vi "Polarization_Simulation.vi"() -> ()   [LabVIEW 2018]
panel:
  in  "Drive Zero Level Down":bool
  in  "Thermally Connect Zero Ensemble":bool
  in  "Zero Ensemble Power":dbl=0.05
  in  "Zero Lorentzian Position":dbl=1.0
  in  "Zero Lorentzian Width":dbl=0.05
  in  "Zero Ensemble Area":dbl=0.1
  in  "Zero Level on":bool
  in  "Gaussian Noise SD":dbl
  in  "AFP Efficiency":dbl=0.8
  in  "Timing (ms)":i32=10
  out "XY Graph 3":cluster{dbl[], "rho- out":dbl[]}[](graph)
  in  "AFP Sweep Direction":u16(ring) items=["Positive", "Negative"]
  in  "RF Proportional to Intensity":bool
  in  "File operation":u16(ring) items=["Open existing file", "Create new file", "Replace existing file"]
  out "XY Graph 2":cluster{"Array":dbl[], "Array 2":dbl[]}(graph)
  in  "Sweep AFP Range":bool
  in  "RF Power":dbl=0.1 min=0.0 max=1.0 step=0.01
  in  "Also use RF Range 2":bool
  in  "RF on":bool
  out "XY Graph":cluster{dbl[], "rho+ array out":dbl[]}[](graph)
  in  "Microwave on":bool
  in  "AFP Slider":cluster{i32, i32}(slide)={0, 500} scale=0.0..500.0
  in  "RF Slider 2":cluster{i32, i32}(slide)={0, 4} scale=0.0..500.0
  in  "RF Slider 1":cluster{i32, i32}(slide)={201, 238} scale=0.0..500.0
  in  "Relaxation Rate":dbl min=0.0 max=1.0 step=0.0001
  in  "Microwave Power":dbl=0.05 min=0.0 max=1.0 step=0.001
  in  "Saturation Polarization":dbl=0.45 min=0.0 max=0.99 step=0.01
  in  "Signal Lorentzian Width":dbl=0.005 min=0.0 step=0.001
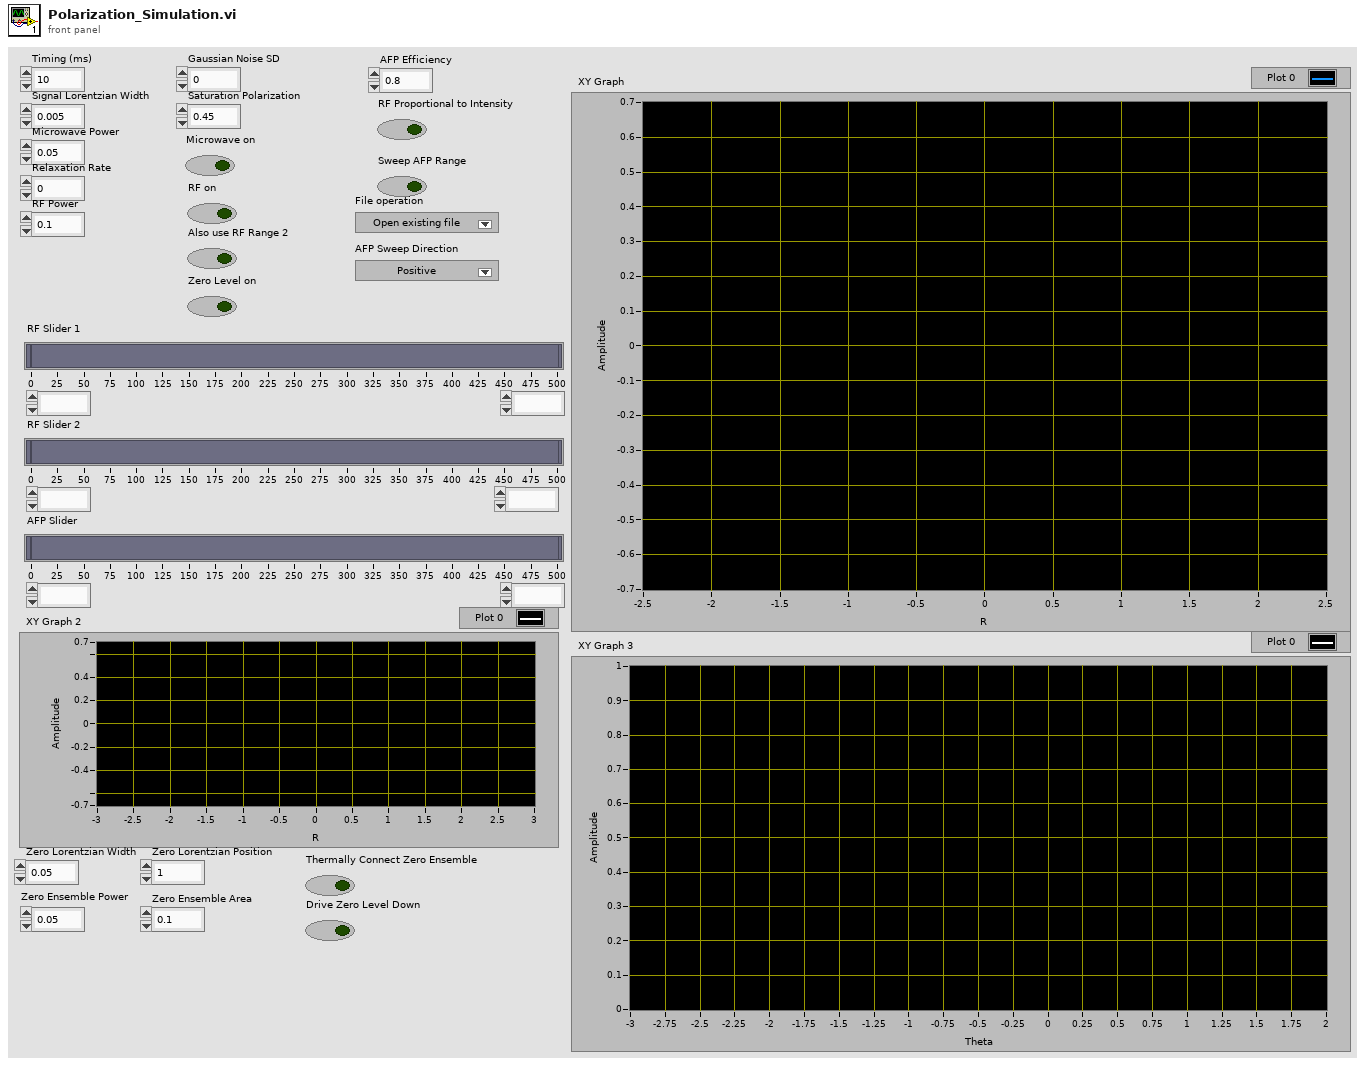
[diagram p1: front panel]
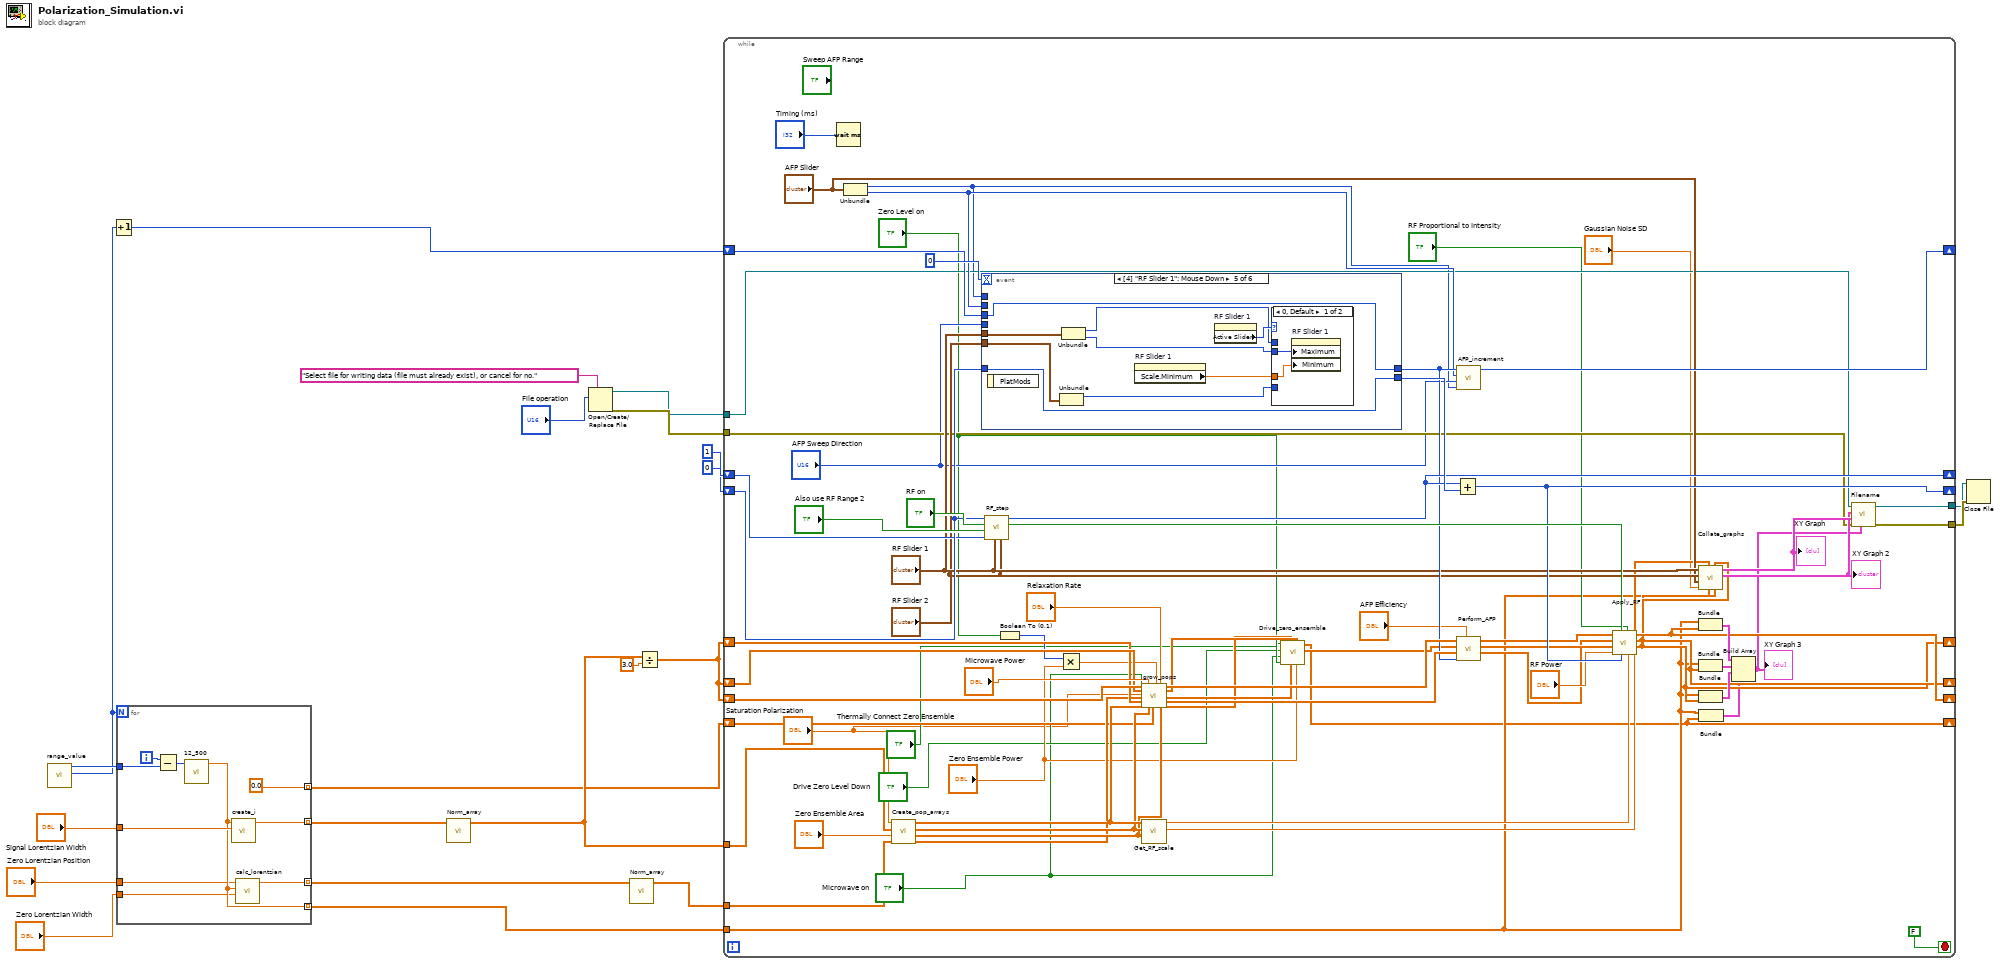
[diagram p0: block diagram]
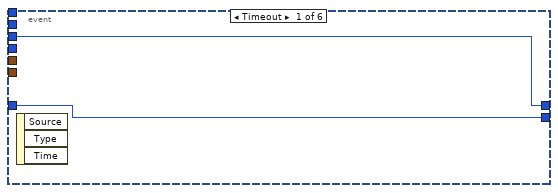
[diagram p2: hidden frame]
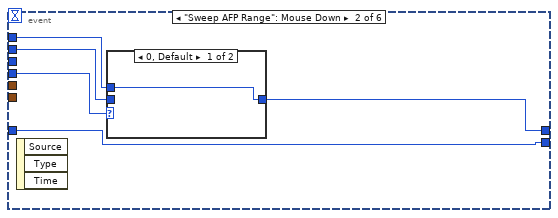
[diagram p3: hidden frame]
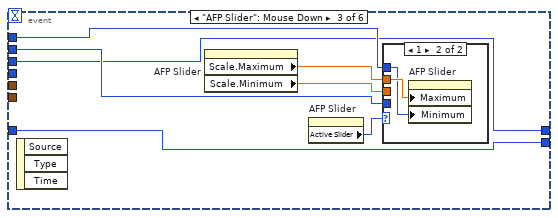
[diagram p5: hidden frame]
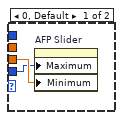
[diagram p6: hidden frame]
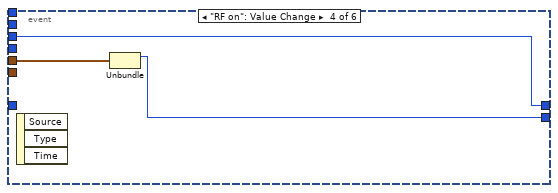
[diagram p7: hidden frame]
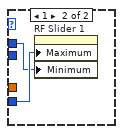
[diagram p8: hidden frame]
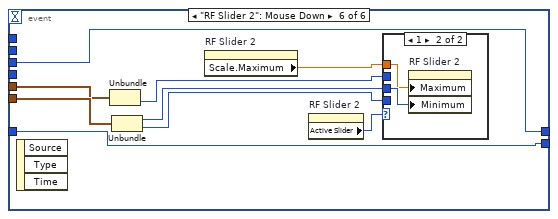
[diagram p9: hidden frame]
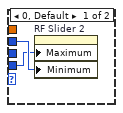
[diagram p10: hidden frame]
diagram:
  n1 = call "range_value.vi"() -> ("NumBins"=w16:i32, "Center"=w22:i32)  [unwired: 10 in]
  n2 = Increment(x=w16) -> (x+1=w15:i32)
  n3 = for {
    N: w16 -> [_]
    tunnel: [w30] -> w20 mode=indexing
    tunnel: w22 -> [w29]
    tunnel: "Signal Lorentzian Width" -> [w28]
    tunnel: [w26] -> w19 mode=indexing
    tunnel: [w27] -> w5 mode=indexing
    tunnel: "Zero Lorentzian Width" -> [w25]
    tunnel: "Zero Lorentzian Position" -> [w24]
    tunnel: [0.0] -> w1 mode=indexing
    i -> [w32]
    n4 = Subtract(x=w32, y=w29) -> (x-y=w31:i32)
    n5 = call "12_500.vi"("Numeric in"=w31) -> ("Numeric out"=w26:dbl)  [unwired: 10 in]
    n6 = call "create_i.vi"("Lorentzian Width"=w28, "Numeric"=w26) -> ("Numeric 2"=w30:dbl)  [unwired: 9 in]
    n7 = call "calc_lorentzian.vi"("Width in"=w25, "x in"=w26, "Position in"=w24) -> ("Value out"=w27:dbl)  [unwired: 8 in]
  }
  n8 = call "Norm_array.vi"("Array"=w20) -> ("Normed Array"=w7:dbl[])  [unwired: 10 in]
  n9 = Open/Create/Replace File(prompt="Select file for writing data (file must already exist), or cancel for no.", operation (0:open)="File operation") -> (refnum out=w12:refnum<file>, error out=w14:errorcluster)  [unwired: 4 in, 1 out]
  n10 = call "Norm_array.vi"("Array"=w5) -> ("Normed Array"=w2:dbl[])  [unwired: 10 in]
  n11 = Divide(x=w7, y=3.0) -> (x/y=w6:dbl[])
  n12 = while {
    tunnel: w7 -> [w103]
    shift-right: [w61] -> _
    shift-left: w6 -> [w100]
    shift-right: [w59] -> _
    shift-left: w6 -> [w98]
    shift-right: [w60] -> _
    shift-left: w6 -> [w99]
    tunnel: w19 -> [w38]
    shift-right: [w90] -> _
    shift-left: 1 -> [w88]
    shift-right: [w92] -> _
    shift-left: 0 -> [w89]
    shift-right: [w86] -> _
    shift-left: w15 -> [w87]
    tunnel: w14 -> [w76]
    tunnel: [w75] -> w13
    tunnel: w12 -> [w74]
    tunnel: [w73] -> w11
    tunnel: w2 -> [w51]
    shift-right: [w37] -> _
    shift-left: w1 -> [w47]
    stop <- FALSE stop-if-true
    n13 = Wait (ms)(milliseconds to wait="Timing (ms)") -> ()  [unwired: 1 out]
    n14 = Unbundle("AFP Slider") -> (w65:i32, w82:i32)
    n15 = call "Create_pop_arrays.vi"("Zero ensemble in"=w51, "Zero ensemble area in"="Zero Ensemble Area", "Normalized I in"=w103, "Saturation Polarization"="Saturation Polarization") -> ("Zero ensemble out"=w50:dbl[], "rho- array out"=w70:dbl[], "rho0 array out"=w71:dbl[], "rho+ array out"=w72:dbl[])  [unwired: 4 in]
    n16 = event shown="[4] \"RF Slider 1\": Mouse Down" {
      selector: _ -> [_ _ _ _ _ _]
      dyn-events: _ -> [_ _ _ _ _ _]
      timeout: 0 -> [_ _ _ _ _ _]
      tunnel: "RF Slider 2" -> [_ _ _ _ w131 w149]
      tunnel: "RF Slider 1" -> [_ _ _ w127 w132 w148]
      tunnel: [w106 w111 w114 w126 w129 w142] -> w93
      tunnel: w89 -> [w106 w111 w114 _ w129 w142]
      tunnel: [w105 w108 w115 w125 w128 w141] -> w83
      tunnel: w87 -> [w105 _ w115 w125 w128 w141]
      tunnel: w65 -> [_ w107 w117 _ _ _]
      tunnel: w82 -> [_ w109 w116 _ _ _]
      tunnel: "AFP Sweep Direction" -> [_ w110 _ _ _ _]
      event Timeout {
        n17 = event-data() -> ()  [unwired: 1 in, 3 out]
      }
      event "Sweep AFP Range": Mouse Down {
        n18 = event-data() -> ()  [unwired: 1 in, 3 out]
        n19 = case shown="0, Default" w110 {
          tunnel: [w112 w113] -> w108
          tunnel: w109 -> [_ w113]
          tunnel: w107 -> [w112 _]
          frame 0, Default {
          }
          frame 1 {
          }
        }
      }
      event "AFP Slider": Mouse Down {
        n20 = event-data() -> ()  [unwired: 1 in, 3 out]
        n21 = property on="AFP Slider" class="Slide (strict)"() -> ("Scale.Maximum"=w119:dbl, "Scale.Minimum"=w118:dbl)  [unwired: 2 in, 2 out]
        n22 = property on="AFP Slider" class="Slide (strict)"() -> ("Active Slider"=w120:i32)  [unwired: 2 in, 2 out]
        n23 = case shown="1" w120 {
          tunnel: w119 -> [_ w124]
          tunnel: w118 -> [w122 _]
          tunnel: w117 -> [_ w123]
          tunnel: w116 -> [w121 _]
          frame 0, Default {
            n24 = property on="AFP Slider" class="Slide (strict)"("Maximum"=w121, "Minimum"=w122) -> ()  [unwired: 2 in, 2 out]
          }
          frame 1 {
            n25 = property on="AFP Slider" class="Slide (strict)"("Maximum"=w124, "Minimum"=w123) -> ()  [unwired: 2 in, 2 out]
          }
        }
      }
      event "RF on": Value Change {
        n26 = event-data() -> ()  [unwired: 1 in, 3 out]
        n27 = Unbundle(w127) -> (w126:i32)  [unwired: 1 out]
      }
      event "RF Slider 1": Mouse Down {
        n28 = event-data() -> ()  [unwired: 1 in, 1 out]
        n29 = Unbundle(w131) -> (w130:i32)  [unwired: 1 out]
        n30 = Unbundle(w132) -> (w135:i32, w134:i32)
        n31 = property on="RF Slider 1" class="Slide (strict)"() -> ("Scale.Minimum"=w133:dbl)  [unwired: 2 in, 2 out]
        n32 = property on="RF Slider 1" class="Slide (strict)"() -> ("Active Slider"=w136:i32)  [unwired: 2 in, 2 out]
        n33 = case shown="0, Default" w136 {
          tunnel: w130 -> [_ w140]
          tunnel: w135 -> [_ w139]
          tunnel: w134 -> [w138 _]
          tunnel: w133 -> [w137 _]
          frame 0, Default {
            n34 = property on="RF Slider 1" class="Slide (strict)"("Maximum"=w138, "Minimum"=w137) -> ()  [unwired: 2 in, 2 out]
          }
          frame 1 {
            n35 = property on="RF Slider 1" class="Slide (strict)"("Maximum"=w140, "Minimum"=w139) -> ()  [unwired: 2 in, 2 out]
          }
        }
      }
      event "RF Slider 2": Mouse Down {
        n36 = event-data() -> ()  [unwired: 1 in, 3 out]
        n37 = Unbundle(w148) -> (w146:i32)  [unwired: 1 out]
        n38 = Unbundle(w149) -> (w144:i32, w145:i32)
        n39 = property on="RF Slider 2" class="Slide (strict)"() -> ("Scale.Maximum"=w143:dbl)  [unwired: 2 in, 2 out]
        n40 = property on="RF Slider 2" class="Slide (strict)"() -> ("Active Slider"=w147:i32)  [unwired: 2 in, 2 out]
        n41 = case shown="1" w147 {
          tunnel: w146 -> [w151 _]
          tunnel: w145 -> [w150 _]
          tunnel: w144 -> [_ w153]
          tunnel: w143 -> [_ w152]
          frame 0, Default {
            n42 = property on="RF Slider 2" class="Slide (strict)"("Maximum"=w150, "Minimum"=w151) -> ()  [unwired: 2 in, 2 out]
          }
          frame 1 {
            n43 = property on="RF Slider 2" class="Slide (strict)"("Maximum"=w152, "Minimum"=w153) -> ()  [unwired: 2 in, 2 out]
          }
        }
      }
    }
    n44 = call "RF_step.vi"("RF Range 2"="RF Slider 2", "RF Range 1"="RF Slider 1", "RF Step Value"=w88, "2 ranges?"="Also use RF Range 2", "RF on"="RF on", "RF Location"=w89) -> ("RF Indicator"=w94:bool, "RF Location out"=w90:i32)  [unwired: 4 in]
    n45 = Boolean To (0,1)(Boolean="Zero Level on") -> (0, 1=w49:i16)
    n46 = Multiply(x=w49, y="Zero Ensemble Power") -> (x*y=w48:dbl)
    n47 = call "grow_pops.vi"("rho+ array"=w100, "rho0 array"=w99, "Sat pol in"="Saturation Polarization", "Zero Ensemble Condition"=w50, "rho- array"=w98, "rho+ condition"=w72, "Microwave power"="Microwave Power", "rho0 condition"=w71, "Microwave on"="Microwave on", "Zero Ensemble Array"=w47, "Zero Level Power"=w48, "Decay rate"="Relaxation Rate", "rho- condition"=w70) -> ("rho+ array out"=w84:dbl[], "rho0 array out"=w46:dbl[], "rho0 decay out"=w45:dbl[], "rho- array out"=w85:dbl[], "Zero Ensemble Out"=w44:dbl[])  [unwired: 2 in]
    n48 = call "Get_RF_scale.vi"("rho-"=w70, "rho0"=w71, "rho+"=w72) -> ("I-  index out"=w68:dbl, "I+ index out"=w69:dbl)  [unwired: 7 in]
    n49 = call "Drive_zero_ensemble.vi"("Zero ensemble power in"="Zero Ensemble Power", "rho0 in"=w46, "rho0 decay in"=w45, "Zero ensemble in"=w44, "Drive Zero Ensemble Up"="Zero Level on", "Microwave on"="Microwave on", "Drive Zero Ensemble Down"="Drive Zero Level Down", "Thermal connection"="Thermally Connect Zero Ensemble") -> ("rho0 out"=w43:dbl[], "Zero ensemble out"=w37:dbl[])  [unwired: 2 in]
    n50 = Add(x=w90, y=w93) -> (x+y=w92:i32)
    n51 = call "AFP_increment.vi"("AFP Min"=w65, "Sweep Direction"="AFP Sweep Direction", "AFP Max"=w82, "AFP Target"=w83) -> ("AFP Target Out"=w86:i32)  [unwired: 7 in]
    n52 = call "Perform_AFP.vi"("AFP Efficiency"="AFP Efficiency", "AFP Target"=w83, "rho-"=w85, "rho0"=w43, "rho+"=w84) -> ("rho- out"=w53:dbl[], "rho0 out"=w54:dbl[], "rho+ out"=w55:dbl[])  [unwired: 4 in]
    n53 = call "Apply_RF.vi"("I- index"=w68, "I+ index"=w69, "RF Proportional to intensity"="RF Proportional to Intensity", "RF Target Position"=w92, "RF indicator"=w94, "RF Power"="RF Power", "rho0"=w54, "rho-"=w53, "rho+"=w55) -> ("rho- out"=w59:dbl[], "rho0 out"=w60:dbl[], "rho+ out"=w61:dbl[])
    n54 = call "Collate_graphs.vi"("R values"=w38, "rho0"=w60, "rho-"=w59, "rho+"=w61, "Gaussian SD in"="Gaussian Noise SD", "AFP Range"="AFP Slider", "RF Range 2"="RF Slider 2", "RF Range 1"="RF Slider 1") -> ("Q Graph"=w77:cluster{"Array":dbl[], "Array 2":dbl[]}, "P Graph and Intensities and RF"=w78:cluster{"Array":dbl[], "Array":dbl[]}[])  [unwired: 2 in]
    "XY Graph" <- w78
    "XY Graph 2" <- w77
    n55 = Bundle(w38, "rho+ out"=w61) -> (w63:cluster{dbl[], "rho+ out":dbl[]})  [unwired: 1 in]
    n56 = Bundle(w38, "rho0 out"=w60) -> (w64:cluster{dbl[], "rho0 out":dbl[]})  [unwired: 1 in]
    n57 = Bundle(w38, "rho- out"=w59) -> (w62:cluster{dbl[], "rho- out":dbl[]})  [unwired: 1 in]
    n58 = Bundle(w38, "Zero ensemble out"=w37) -> (w36:cluster{dbl[], "Zero ensemble out":dbl[]})  [unwired: 1 in]
    n59 = Build Array(w63, w64, w62, w36) -> (w35:cluster{dbl[], "Zero ensemble out":dbl[]}[])
    "XY Graph 3" <- w35
    n60 = call "Filename.vi"("Densities and De Boer"=w35, "error in (no error)"=w76, "P Graph and Intensities and RF"=w78, "Q Graph"=w77, "Byte Stream File in"=w74) -> ("error out"=w75:errorcluster, "Byte Stream File out"=w73:refnum<file>)  [unwired: 5 in]
  }
  n61 = Close File(refnum=w11, error in=w13) -> ()  [unwired: 2 out]
